vi "Set Value.vi"(8 "error in (no error)":errorcluster, 10 "Project Info Value":string, 11 "String Item Configuration in":refnum<class "String Item Configuration.lvclass">) -> (0 "error out":errorcluster, 3 "String Item Configuration out":refnum<class "String Item Configuration.lvclass">)   [LabVIEW 2013, in "Item Configuration.lvlib" / "String Item Configuration.lvclass"]
uses:
  String Item Configuration.lvclass
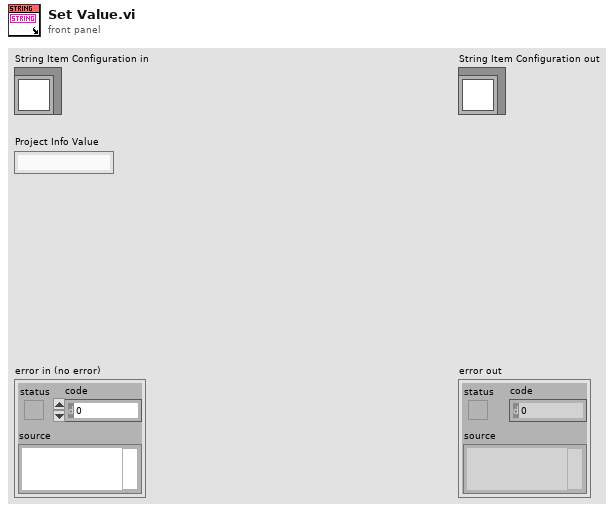
[diagram p1: front panel]
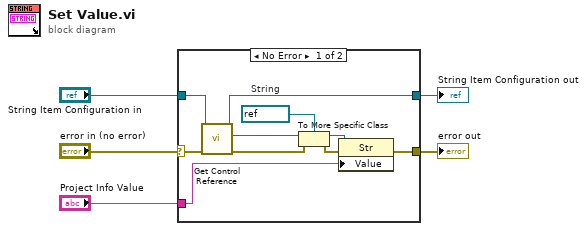
[diagram p0: block diagram]
diagram:
  n1 = case shown="No Error" "error in (no error)" {
    selector: "error in (no error)" -> [w12 w17]
    tunnel: [w13 w17] -> w2
    tunnel: "String Item Configuration in" -> [w11 w16]
    tunnel: [w10 w16] -> w1
    tunnel: "Project Info Value" -> [w6 _]
    frame No Error {
      w14 = refnum<vi> refnum  # String
      n2 = call-dynamic "Get Control Reference.vi"("error in (no error)"=w12, "Item Configuration in"=w11) -> ("error out"=w9:errorcluster, "Control Reference"=w15:refnum<vi>, "Item Configuration out"=w10:refnum<class "String Item Configuration.lvclass">)  [unwired: 7 in]
      n3 = To More Specific Class(target class=w14, reference=w15, error in=w9) -> (specific class reference=w7:refnum<vi>, error out=w8:errorcluster)
      n4 = property class="Str"(reference=w7, error in=w8, "Value"=w6) -> (error out=w13:errorcluster)  [unwired: 1 out]
    }
    frame Error {
    }
  }
  "error out" <- w2
  "String Item Configuration out" <- w1
